vi "Transmitter_Example.vi"() -> ()   [LabVIEW 2022 SP3]
uses:
  <instrlib>/niUSRP/niUSRP Write Tx Data (CDB Cluster).vi
panel:
  in  "String Critical Data 2":string="Critical Dataaaaa\nCritical Dataaaaa\nCritical Dataaaaa\nCritical Dataaaaa\nCritical Dataaaaa\nNon Critical Data\nNon Critical Data\nNon Critical Data\nNon Critical Data\nNon Critical Data"
  in  "milliseconds to wait":u32=100
  in  "OFDM 4QAM / 16QAM":bool
  out "AuxString 2":string
  out "AuxString":string
  in  "Previous Button":bool caption="Both Critical and Non Critical\nData must be equal size."
  in  "New Critical Data":string="Non Critical Data\nNon Critical Data\nNon Critical Data\nNon Critical Data\nNon Critical Data"
  in  "New Non Critical Data":string="Critical Dataaaaa\nCritical Dataaaaa\nCritical Dataaaaa\nCritical Dataaaaa\nCritical Dataaaaa"
  out "Frame Duration 2":dbl format="%#_6p"
  in  "Alpha":dbl=0.05 min=0.0 max=1.0 step=0.05
  out "Bits length 2":i32
  in  "String Critical Data":string="Non Critical Data\nNon Critical Data\nNon Critical Data\nNon Critical Data\nNon Critical Data"
  in  "Modulation parameter":T1
  out "Bits length":i32
  out "Frame Duration":dbl format="%#_6p"
  out "Waveform Graph":cluster{"t0":dbl, "dt":dbl, "Y":dbl[]}(graph)
  in  "stop":bool
  in  "String Non Critical Data":string="Critical Dataaaaa\nCritical Dataaaaa\nCritical Dataaaaa\nCritical Dataaaaa\nCritical Dataaaaa"
  out "USRP CoercedParamters":T2={"coerced IQ rate"=100000.0, "coerced carrier frequency"=100000.0, "coerced gain"=0.0} {"coerced gain" format="%#_6f"; "coerced carrier frequency" format="%#_6p"; "coerced IQ rate" format="%#_6p"}
  out "error out":errorcluster
  in  "error in (no error)":errorcluster
  in  "USRP ControledParameters":T3={"active antenna"="TX1", "gain"=10.0, "carrier frequency"=2400000000.0, "IQ rate"=2000000.0} {"IQ rate" format="%#_6p"; "carrier frequency" format="%#_6p"; "gain" format="%#_6f"}
  in  "device names":refnum<k15>="RIO0"
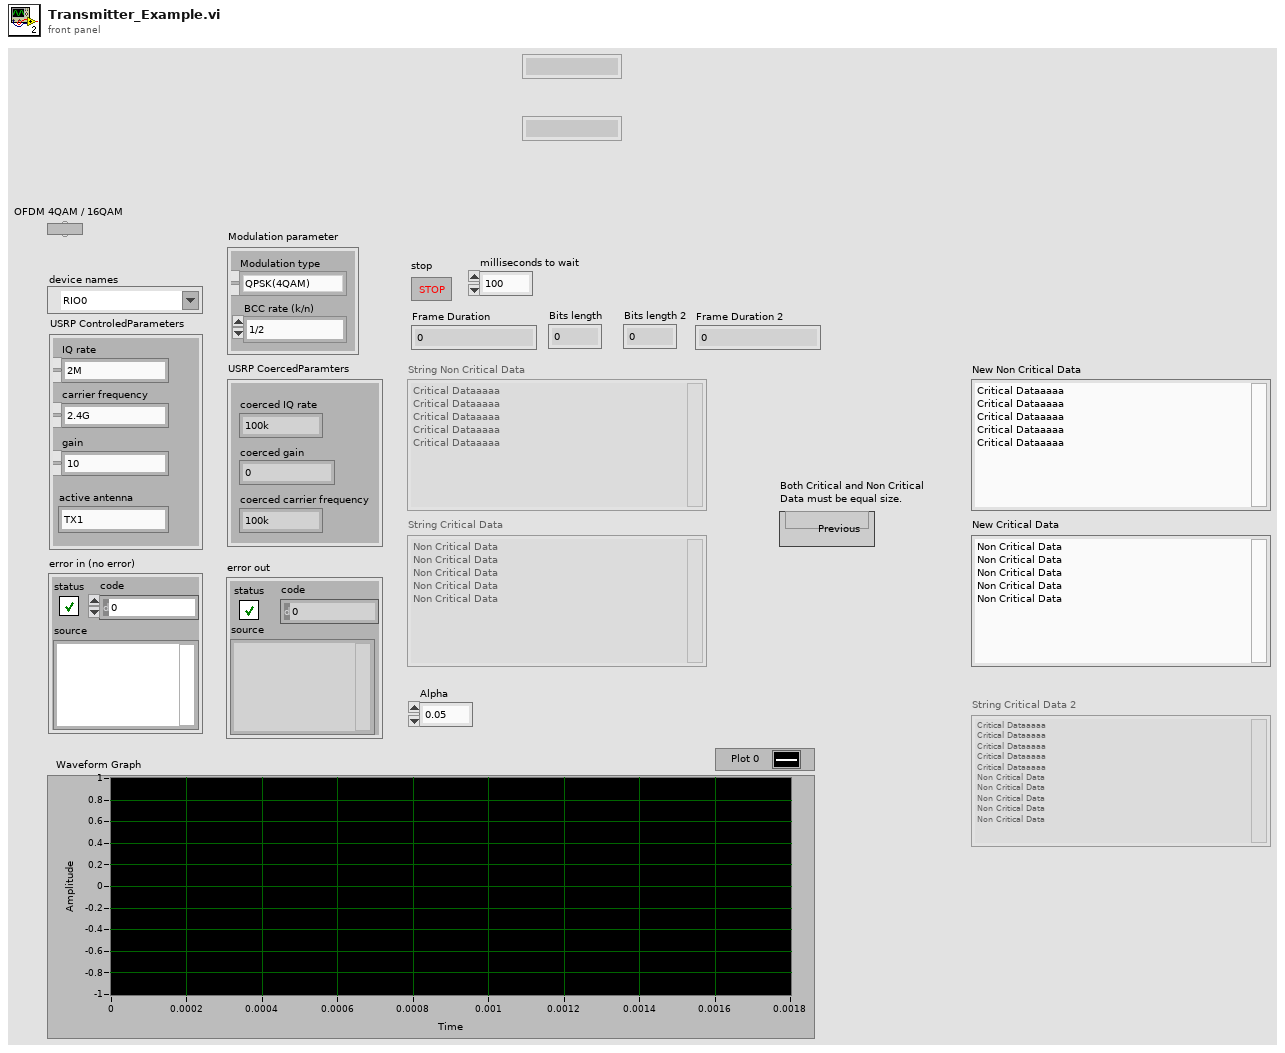
[diagram p1: front panel]
types:
  T1 = cluster{"Modulation type":enum16{"QPSK(4QAM)", "64QAM", "16QAM", "BPSK"}, "BCC rate (k/n)":enum16{"1/2", "2/3", "3/4"}}
  T2 = cluster{"coerced IQ rate":dbl, "coerced carrier frequency":dbl, "coerced gain":dbl}
  T3 = cluster{"active antenna":string, "gain":dbl, "carrier frequency":dbl, "IQ rate":dbl}
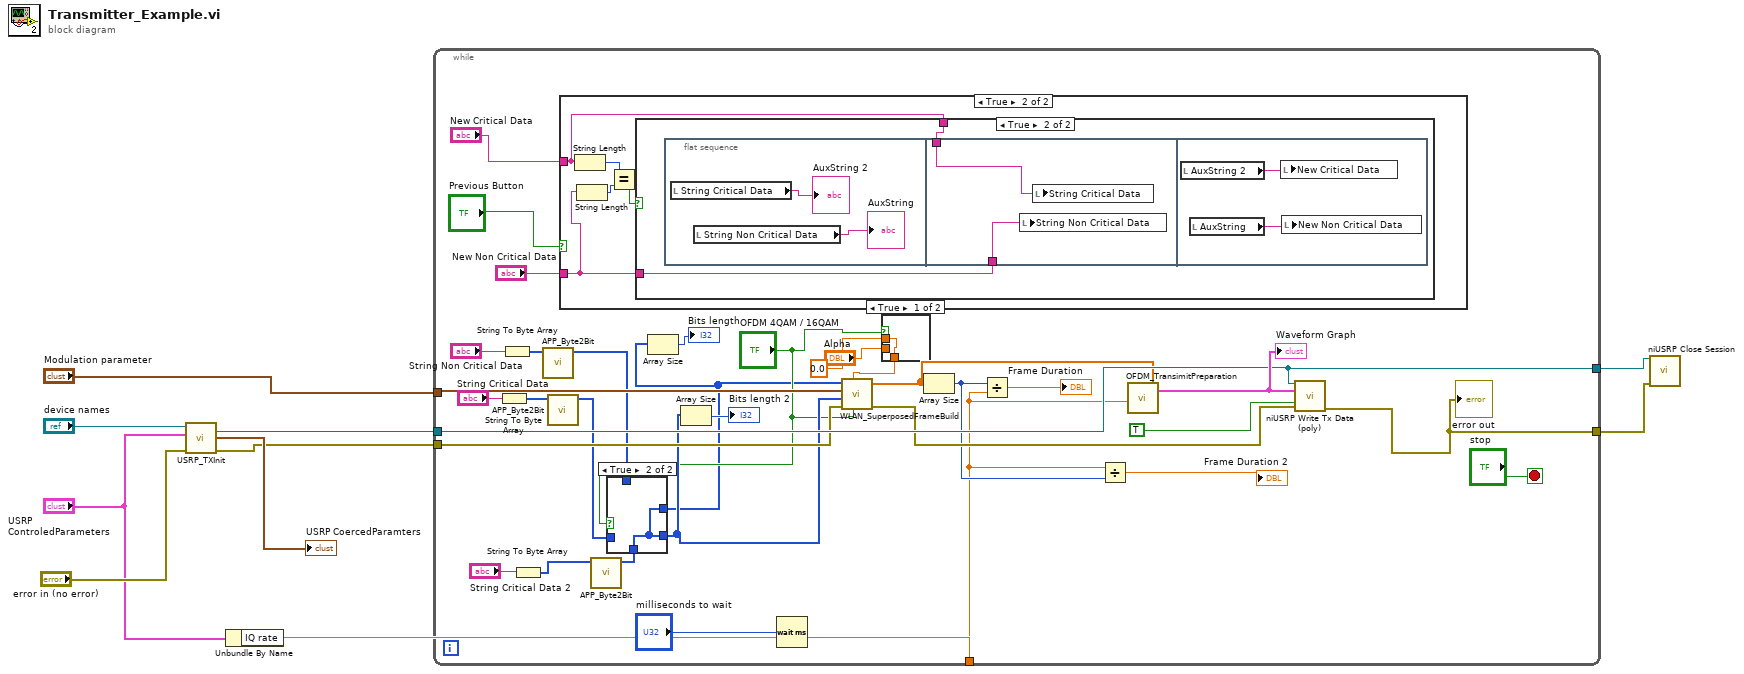
[diagram p0: block diagram]
diagram:
  n1 = call "USRP_TXInit.vi"("device names"="device names", "USRP ControledParameters"="USRP ControledParameters", "error in (no error)"="error in (no error)") -> ("session handle out"=w8:refnum<k15>, "USRP CoercedParamters"=→"USRP CoercedParamters":T2, "error out"=w4:errorcluster)  [unwired: 5 in]
  n2 = Unbundle By Name("USRP ControledParameters") -> ("IQ rate"=w1:dbl)
  n3 = while {
    tunnel: w8 -> [w39]
    tunnel: "Modulation parameter" -> [w34]
    tunnel: w4 -> [w33]
    tunnel: w1 -> [w29]
    tunnel: [w39] -> w3
    tunnel: [w38] -> w2
    stop <- "stop" stop-if-true
    n4 = String To Byte Array(string="String Critical Data") -> (unsigned byte array=w35:u8[])
    n5 = String To Byte Array(string="String Non Critical Data") -> (unsigned byte array=w36:u8[])
    n6 = String To Byte Array(string="String Critical Data 2") -> (unsigned byte array=w17:u8[])
    n7 = call "APP_Byte2Bit.vi"("input byte stream"=w36) -> ("output bit stream"=w12:i8[])  [unwired: 10 in]
    n8 = call "APP_Byte2Bit.vi"("input byte stream"=w35) -> ("output bit stream"=w15:i8[])  [unwired: 10 in]
    n9 = case shown="True" "Previous Button" {
      tunnel: "New Non Critical Data" -> [_ w54]
      tunnel: "New Critical Data" -> [_ w50]
      frame False {
      }
      frame True {
        n10 = String Length(string=w50) -> (length=w53:i32)
        n11 = String Length(string=w54) -> (length=w52:i32)
        n12 = Equal?(x=w53, y=w52) -> (x = y?=w51:bool)
        n13 = case shown="True" w51 {
          tunnel: w54 -> [_ w56]
          tunnel: w50 -> [_ w55]
          frame False {
          }
          frame True {
            n14 = flat-sequence {
              tunnel: w56 -> [w60]
              tunnel: w55 -> [w59]
              frame #0 {
                n15 = local read "String Critical Data"() -> (→"AuxString 2":string)
                n16 = local read "String Non Critical Data"() -> (→"AuxString":string)
              }
              frame #1 {
                n17 = local write "String Non Critical Data"(w60) -> ()
                n18 = local write "String Critical Data"(w59) -> ()
              }
              frame #2 {
                n19 = local read "AuxString 2"() -> (w61:string)
                n20 = local read "AuxString"() -> (w62:string)
                n21 = local write "New Critical Data"(w61) -> ()
                n22 = local write "New Non Critical Data"(w62) -> ()
              }
            }
          }
        }
      }
    }
    n23 = call "APP_Byte2Bit.vi"("input byte stream"=w17) -> ("output bit stream"=w14:i8[])  [unwired: 10 in]
    n24 = case shown="True" "OFDM 4QAM / 16QAM" {
      tunnel: [w46 w47] -> w16
      tunnel: w15 -> [w46 _]
      tunnel: w14 -> [_ w47]
      tunnel: [w45 w47] -> w11
      tunnel: w12 -> [w45 _]
      frame False {
      }
      frame True {
      }
    }
    n25 = Array Size(array=w11) -> (size(s)=→"Bits length":i32)
    n26 = Array Size(array=w16) -> (size(s)=→"Bits length 2":i32)
    n27 = Wait (ms)(milliseconds to wait="milliseconds to wait") -> ()  [unwired: 1 out]
    n28 = case shown="True" "OFDM 4QAM / 16QAM" {
      tunnel: [w48 w49] -> w22
      tunnel: "Alpha" -> [_ w49]
      tunnel: 0.0 ("Alpha 2") -> [w48 _]
      frame True {
      }
      frame False {
      }
    }
    n29 = call "WLAN_SuperposedFrameBuild.vi"("OFDMON"="OFDM 4QAM / 16QAM", "Alpha"=w22, "error in (no error)"=w33, "data in 2"=w16, "Modulation parameter"=w34, "data in"=w11) -> ("error out"=w32:errorcluster, "output array"=w31:cdb[])  [unwired: 4 in]
    n30 = Array Size(array=w31) -> (size(s)=w30:i32)
    n31 = Divide(x=w30, y=w29) -> (x/y=→"Frame Duration":dbl)
    n32 = Divide(x=w29, y=w30) -> (x/y=→"Frame Duration 2":dbl)
    n33 = call "OFDM_TransimitPreparation.vi"("IQ rate"=w29, "array"=w31) -> ("output cluster"=w41:cluster{"t0":dbl, "dt":dbl, "Y":cdb[]})  [unwired: 9 in]
    "Waveform Graph" <- w41
    n34 = call-poly <instrlib>:"niUSRP Write Tx Data (poly).vi"("session handle"=w39, "data"=w41, "end of data?"=TRUE, "error in (no error)"=w32) -> ("error out"=w38:errorcluster)  [unwired: 10 in, 1 out]
    "error out" <- w38
  }
  n35 = call <instrlib>:"niUSRP Close Session.vi"("session handle"=w3, "error in (no error)"=w2) -> ()  [unwired: 13 in, 1 out]
